vi "InitApplication.vi"(8 "error in (no error)":errorcluster, 10 "Application Data in":T2, 11 "GUI Refs":T1) -> (0 "error out":errorcluster)   [LabVIEW 2019]
uses:
  Typedefs/#cluster_ApplicationData.ctl
  Typedefs/Acquisition Thread/#cluster_AcqQueueData.ctl
  Typedefs/Acquisition Thread/#enum_AcquisitionTask.ctl
  Typedefs/Saving Thread/#cluster_SavingQueueData.ctl
  Typedefs/Saving Thread/#enum_SavingTask.ctl
  <vilib>/ActorFramework/Message Enqueuer/Message Enqueuer.lvclass
  Typedefs/#cluster_GUIRefs.ctl
  Application Configuration VIs/#enum_FGVAction.ctl
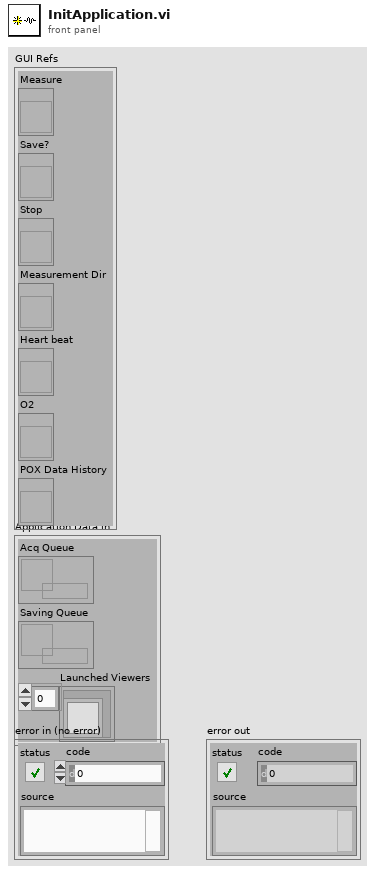
[diagram p1: front panel]
types:
  T1 = typedef "#cluster_GUIRefs.ctl" = cluster{"Measure":refnum<vi>, "Save?":refnum<vi>, "Stop":refnum<vi>, "Measurement Dir":refnum<vi>, "Heart beat":refnum<vi>, "O2":refnum<vi>, "POX Data History":refnum<vi>}
  T2 = typedef "#cluster_ApplicationData.ctl" = cluster{"Acq Queue":refnum<queue>, "Saving Queue":refnum<queue>, "Launched Viewers":refnum<class "Message Enqueuer.lvclass">[]}
  T3 = typedef "#enum_FGVAction.ctl" = enum16{"Get", "Set"}
  T4 = typedef "#cluster_AcqQueueData.ctl" = cluster{"Task":T5, "Data":variant}
  T5 = typedef "#enum_AcquisitionTask.ctl" = enum16{"Init", "Start", "Finish", "Close"}
  T6 = typedef "#cluster_AppConfiguration.ctl" = cluster{"Measurements Directory":path}
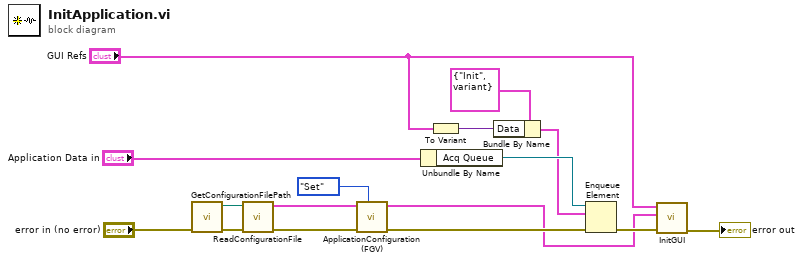
[diagram p0: block diagram]
diagram:
  n1 = call "GetConfigurationFilePath.vi"() -> ("Configuration File Path"=w5:path)  [unwired: 11 in]
  n2 = call "ReadConfigurationFile.vi"("Error in"="error in (no error)", "Configuration File Path"=w5) -> ("Error out"=w6:errorcluster, "App Configuration"=w3:T6)  [unwired: 8 in]
  n3 = call "ApplicationConfiguration (FGV).vi"("FGV Action"=#enum_FGVAction."Set", "Error in"=w6, "App Configuration in"=w3) -> ("Error out"=w4:errorcluster, "App Configuration out"=w1:T6)  [unwired: 7 in]
  n4 = Unbundle By Name("Application Data in") -> ("Acq Queue"=w9:refnum<queue>)
  n5 = To Variant(anything="GUI Refs") -> (Variant=w12:variant)
  n6 = Bundle By Name(cluster=T4 {"Task"=enum."Init", "Data"=variant} ("Acq Data"), "Data"=w12) -> (w8:T4)
  n7 = Enqueue Element(queue=w9, element=w8, error in (no error)=w4) -> (error out=w7:errorcluster)  [unwired: 1 in, 2 out]
  n8 = call "InitGUI.vi"("error in (no error)"=w7, "App Configuration"=w1, "GUI Refs"="GUI Refs") -> ("error out"=→"error out":errorcluster)  [unwired: 8 in]
